vi "update controls.vi"(6 "selectors":T1, 8 "error in (no error)":errorcluster, 9 "plan section":string, 10 "vi name":string, 11 "vi ref in":refnum<vi>) -> (0 "error out":errorcluster, 3 "vi ref out":refnum<vi>)   [LabVIEW 2024, in "controls manager.lvlib"]
uses:
  controls manager.lvlib
  selectors.ctl
  fgv actions.ctl
  <vilib>/Utility/error.llb/Error Cluster From Error Code.vi
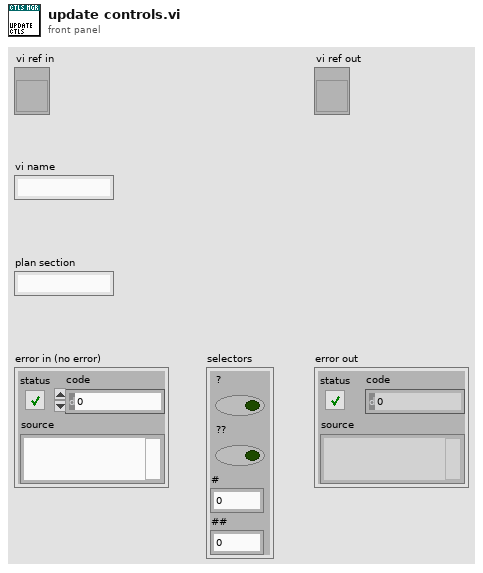
[diagram p1: front panel]
types:
  T1 = typedef "controls manager.lvlib/selectors.ctl" = cluster{"?":bool, "??":bool, "#":u16, "##":u16}
  T2 = typedef "controls manager.lvlib/fgv actions.ctl" = enum16{"create", "get", "destroy"}
  T3 = typedef "controls manager.lvlib/collection type.ctl" = map{string, T4}
  T4 = typedef "controls manager.lvlib/entry type.ctl" = cluster{"controls":map{string, T5}, "plan":T6}
  T5 = typedef "controls manager.lvlib/control.ctl" = cluster{"refnum":refnum<vi>, "index":i32}
  T6 = typedef "controls manager.lvlib/controls plan.ctl" = map{string, T7[]}
  T7 = typedef "controls manager.lvlib/key value pair.ctl" = cluster{"key":string, "value":string}
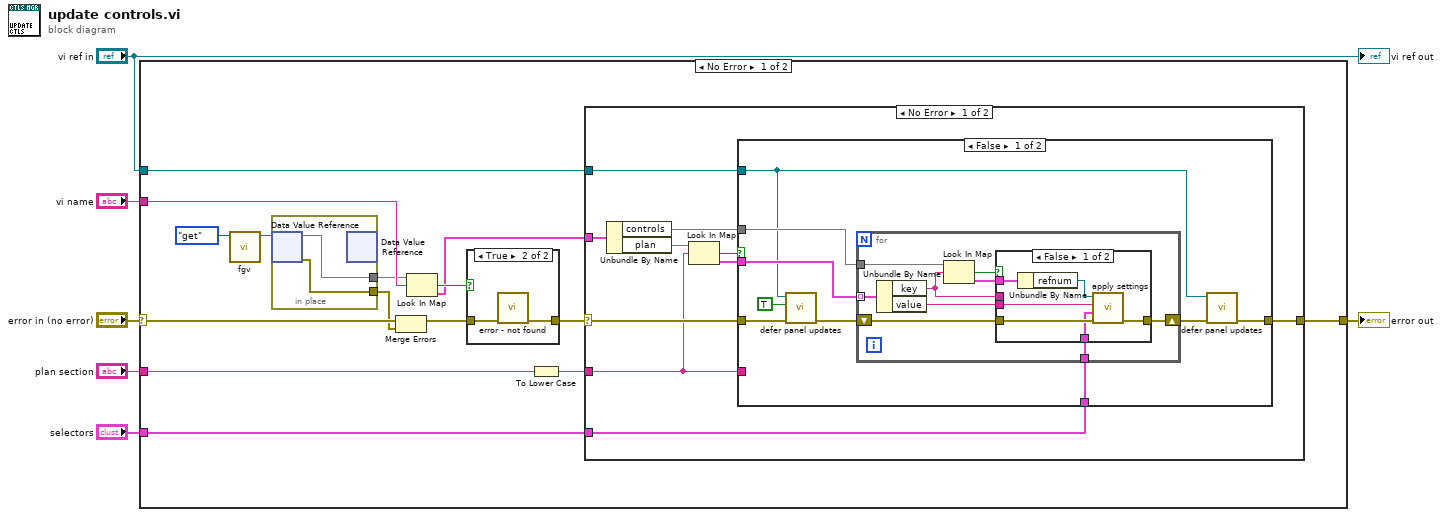
[diagram p0: block diagram]
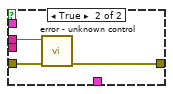
[diagram p2: hidden frame]
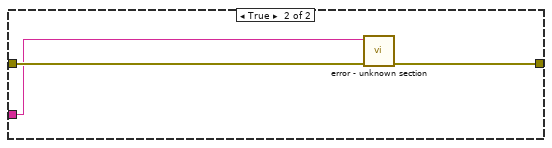
[diagram p3: hidden frame]
diagram:
  n1 = case shown="No Error" "error in (no error)" {
    selector: "error in (no error)" -> [w16 w68]
    tunnel: "vi ref in" -> [w20 _]
    tunnel: "selectors" -> [w19 _]
    tunnel: "vi name" -> [w18 _]
    tunnel: [w17 w68] -> w4
    tunnel: "plan section" -> [w14 _]
    frame No Error {
      n2 = call "fgv.vi"("action"=fgv_actions."get") -> ("dvr"=w8:refnum<data-value>)  [unwired: 9 in, 1 out]
      n3 = in-place {
        in-place-border: [w67] -> w11
        in-place-border: [w66] -> w10
        n4 = in-place-dvr #1(w8) -> (w67:T3, w66:errorcluster)
        n5 = in-place-dvr #1() -> ()  [unwired: 1 in, 2 out]
      }
      n6 = Merge Errors(w16, w10) -> (w13:errorcluster)
      n7 = Look In Map(map=w11, key=w18) -> (key not found?=w12:bool, value=w7:T4)  [unwired: 1 in]
      n8 = case shown="True" w12 {
        tunnel: w13 -> [w63 w65]
        tunnel: [w63 w64] -> w15
        frame False {
        }
        frame True {
          n9 = call "error - not found.vi"("error in (no error)"=w65) -> ("error out"=w64:errorcluster)  [unwired: 10 in]
        }
      }
      n10 = To Lower Case(string=w14) -> (all lower case string=w21:string)
      n11 = case shown="No Error" w15 {
        selector: w15 -> [w31 w62]
        tunnel: w7 -> [w30 _]
        tunnel: w21 -> [w23 _]
        tunnel: [w25 w62] -> w17
        tunnel: w19 -> [w24 _]
        tunnel: w20 -> [w22 _]
        frame No Error {
          n12 = Unbundle By Name(w30) -> ("controls"=w26:map{string, T5}, "plan"=w29:T6)
          n13 = Look In Map(map=w29, key=w23) -> (key not found?=w28:bool, value=w27:T7[])  [unwired: 1 in]
          n14 = case shown="False" w28 {
            tunnel: w27 -> [w40 _]
            tunnel: w26 -> [w39 _]
            tunnel: [w33 w60] -> w25
            tunnel: w31 -> [w37 w61]
            tunnel: w24 -> [w36 _]
            tunnel: w23 -> [_ w59]
            tunnel: w22 -> [w32 _]
            frame False {
              n15 = call "defer panel updates.vi"("error in (no error)"=w37, "defer? (F)"=TRUE, "vi ref"=w32) -> ("error out"=w35:errorcluster)  [unwired: 8 in]
              n16 = for {
                tunnel: w40 -> [w49] mode=indexing
                tunnel: w39 -> [w48]
                shift-right: [w44] -> w38
                shift-left: w35 -> [w43]
                tunnel: w36 -> [w42]
                n17 = Unbundle By Name(w49) -> ("key"=w41:string, "value"=w45:string)
                n18 = Look In Map(map=w48, key=w41) -> (key not found?=w46:bool, value=w47:T5)  [unwired: 1 in]
                n19 = case shown="False" w46 {
                  tunnel: w47 -> [w51 _]
                  tunnel: w45 -> [w55 _]
                  tunnel: [w54 w57] -> w44
                  tunnel: w43 -> [w53 w58]
                  tunnel: w42 -> [w52 _]
                  tunnel: w41 -> [_ w56]
                  frame False {
                    n20 = Unbundle By Name(w51) -> ("refnum"=w50:refnum<vi>)
                    n21 = call "apply settings.vi"("error in (no error)"=w53, "selectors"=w52, "settings"=w55, "refnum"=w50) -> ("error out"=w54:errorcluster)  [unwired: 7 in]
                  }
                  frame True {
                    n22 = call "error - unknown control.vi"("error in (no error)"=w58, "label"=w56) -> ("error out"=w57:errorcluster)  [unwired: 9 in]
                  }
                }
              }
              n23 = call "defer panel updates.vi"("error in (no error)"=w38, "vi ref"=w32) -> ("error out"=w33:errorcluster)  [unwired: 9 in]
            }
            frame True {
              n24 = call "error - unknown section.vi"("error in (no error)"=w61, "section"=w59) -> ("error out"=w60:errorcluster)  [unwired: 9 in]
            }
          }
        }
        frame Error {
        }
      }
    }
    frame Error {
    }
  }
  "error out" <- w4
  "vi ref out" <- "vi ref in"
